vi "Test Get Named Ranges.vi"(11 "Test Case In":refnum<class "Test Open Xml.lvclass">) -> (0 "error out":errorcluster, 3 "Test Case Out":refnum<class "Test Open Xml.lvclass">)   [LabVIEW 2020, in "Test Open Xml.lvclass"]
uses:
  Test Open Xml.lvclass
  C:/Program Files/National Instruments/LabVIEW 2025/vi.lib/Astemes/LUnit/Test Case.lvclass
  Source/Cell DataType.ctl
  <vilib>/Astemes/LUnit/Test Case.lvclass/Test Case.ctl
  75fec585-59d7-4050-a2b8-3c2cca1562a1.vi
  c842f118-240e-4daf-a2da-7e37ae4209a2.vi
  f6172169-f5fa-494e-af90-d316b3356897.vi
  a79cc3df-4eee-4479-a611-92cfecdf73e7.vi
  c842f118-240e-4daf-a2da-7e37ae4209a2.vi/492de82e-1417-411c-9e2f-039d34dd0f56.vi
  Source/Excel Cell Address to Numeric Indices.vi
  Source/Numeric Indices to Excel Cell Address.vi
  c842f118-240e-4daf-a2da-7e37ae4209a2.vi/b0ca85c4-5697-48fb-9b3b-38ca6a246b1e.vi
  <vilib>/Astemes/LUnit/Append Fail Result.vi
  <vilib>/Astemes/LUnit/Append Pass Result.vi
  <vilib>/Astemes/LUnit/Run In UI.vi
  <vilib>/Utility/error.llb/Clear Errors.vi
  Source/Get WorksheetPart.vi
  Source/Get or Add Cell.vi
  Source/Create CellValue.vi
  Source/Set CellValue.vi
  Source/Set Cell DataType.vi
  Source/Open Xml.lvlib
  <vilib>/Astemes/LUnit/Test Case.lvclass
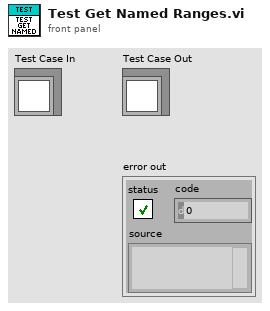
[diagram p1: front panel]
types:
  T1 = enum16{"Boolean", "Numeric", "String", "String2", "Array"}
  T2 = enum16{"Boolean", "Numeric", "String", "String2", "Array"}[]
  T3 = typedef "Open Xml.lvlib/Cell DataType.ctl" = enum16{"Void", "Boolean", "Number", "Error", "SharedString", "String", "InlineString", "Date"}
  T4 = cluster{"Number":dbl, "String":string, "Boolean":bool, "Timestamp":timestamp, "Error":errorcluster}
  T5 = cluster{"Number":dbl, "String":string, "Boolean":bool, "Time Stamp":timestamp, "Error":errorcluster}[][]
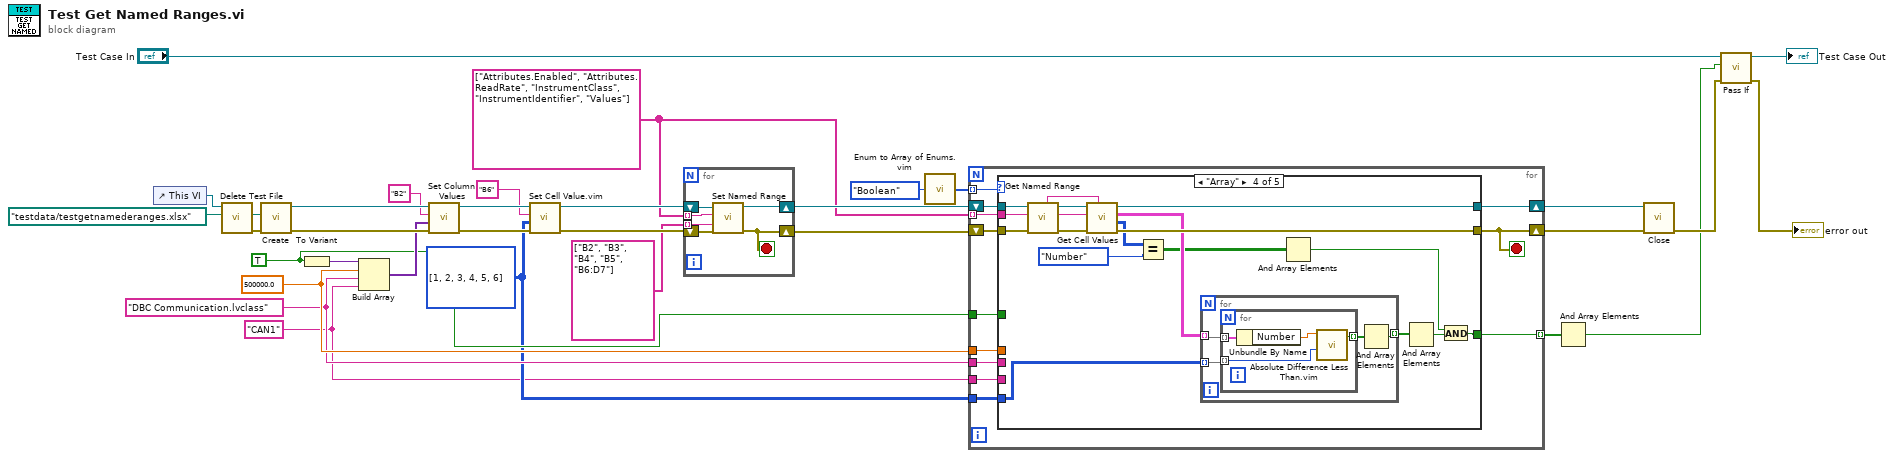
[diagram p0: block diagram]
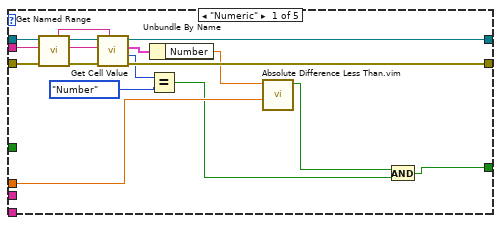
[diagram p2: hidden frame]
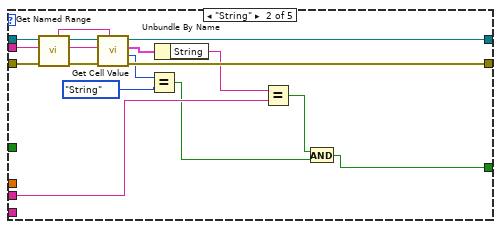
[diagram p3: hidden frame]
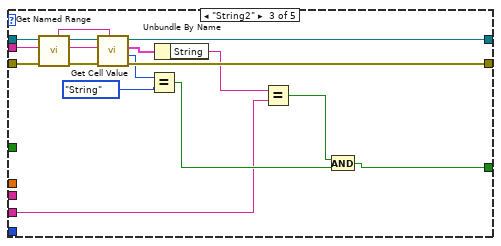
[diagram p4: hidden frame]
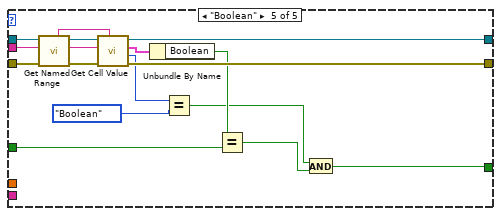
[diagram p5: hidden frame]
diagram:
  w4 = i32[][] [[1, 2, 3], [4, 5, 6]]
  w1 = "CAN1" ("element")
  w5 = "DBC Communication.lvclass"
  w7 = 500000.0
  w6 = TRUE
  w11 = string[] ["Attributes.Enabled", "Attributes.ReadRate", "InstrumentClass", "InstrumentIdentifier", "Values"] ("Range Names")
  n1 = control-ref of="This VI"() -> (w28:refnum<vi>)
  n2 = call "Delete Test File.vi"("name or relative path"=path "testdata/testgetnamederanges.xlsx", "VI in"=w28) -> ("error out"=w25:errorcluster, "deleted path"=w26:path)  [unwired: 8 in]
  n3 = call "Create.vi"("error in"=w25, "Path"=w26) -> ("error out"=w24:errorcluster, "SpreadsheetDoc"=w22:refnum<k24>)  [unwired: 8 in]
  n4 = To Variant(anything=w6) -> (Variant=w19:variant)
  n5 = Build Array(w19, w7, w5, w1) -> (w20:variant[])
  n6 = call "Set Column Values.vi"("error in"=w24, "Values"=w20, "Cell Address"="B2", "SpreadsheetDoc"=w22) -> ("error out"=w23:errorcluster, "SpreadsheetDoc out"=w16:refnum<k24>)  [unwired: 6 in]
  n7 = call "Set Cell Value.vim"("error in"=w23, "Value"=w4, "Cell Address"="B6", "SpreadsheetDoc in"=w16) -> ("error out"=w17:errorcluster, "SpreadsheetDoc out"=w15:refnum<k24>)  [unwired: 6 in]
  n8 = for {
    tunnel: w11 -> [w37] mode=indexing
    tunnel: string[] ["B2", "B3", "B4", "B5", "B6:D7"] ("Range Names") -> [w36] mode=indexing
    shift-right: [w35] -> w18
    shift-left: w17 -> [w39]
    shift-right: [w34] -> w12
    shift-left: w15 -> [w38]
    stop <- w35 stop-if-true
    n9 = call "Set Named Range.vi"("error in"=w39, "Cell Range"=w36, "Named Range Identifier"=w37, "SpreadsheetDoc in"=w38) -> ("error out"=w35:errorcluster, "SpreadsheetDoc out"=w34:refnum<k24>)  [unwired: 6 in]
  }
  n10 = call "Enum to Array of Enums.vim"("enum"=T1."Boolean") -> ("array of enums"=w8:T2)
  n11 = for {
    shift-right: [w47] -> w30
    shift-left: w18 -> [w51]
    tunnel: w11 -> [w50] mode=indexing
    shift-right: [w48] -> w10
    shift-left: w12 -> [w49]
    tunnel: w8 -> [w46] mode=indexing
    tunnel: w7 -> [w45]
    tunnel: w6 -> [w44]
    tunnel: w5 -> [w43]
    tunnel: w4 -> [w42]
    tunnel: [w41] -> w3 mode=indexing
    tunnel: w1 -> [w40]
    stop <- w47 stop-if-true
    n12 = case shown="\"Array\"" w46 {
      tunnel: w51 -> [w67 w84 w101 w119 w144]
      tunnel: w50 -> [w66 w83 w100 w118 w143]
      tunnel: w49 -> [w65 w82 w99 w117 w142]
      tunnel: [w64 w81 w98 w116 w141] -> w48
      tunnel: [w60 w77 w94 w112 w137] -> w47
      tunnel: w45 -> [w55 _ _ _ _]
      tunnel: w44 -> [_ _ _ _ w132]
      tunnel: w43 -> [_ w72 _ _ _]
      tunnel: w42 -> [_ _ _ w109 _]
      tunnel: [w52 w69 w87 w105 w129] -> w41
      tunnel: w40 -> [_ _ w86 _ _]
      frame "Numeric" {
        n13 = call "Get Named Range.vi"("error in"=w67, "Range Identifier"=w66, "SpreadsheetDoc in"=w65) -> ("error out"=w68:errorcluster, "Range"=w63:string, "SpreadsheetDoc out"=w62:refnum<k24>, "Sheet Name"=w61:string)  [unwired: 5 in]
        n14 = call "Get Cell Value.vi"("Sheet Name"=w61, "error in"=w68, "Cell Address"=w63, "SpreadsheetDoc in"=w62) -> ("error out"=w60:errorcluster, "Type"=w58:T3, "Cell Value"=w59:T4, "SpreadsheetDoc out"=w64:refnum<k24>)  [unwired: 4 in]
        n15 = Equal?(x=w58, y=Cell_DataType."Number") -> (x = y?=w54:bool)
        n16 = Unbundle By Name(w59) -> ("Number"=w56:dbl)
        n17 = call "Absolute Difference Less Than.vim"("Number 2"=w55, "Number 1"=w56) -> ("In Limit"=w53:bool)  [unwired: 9 in]
        n18 = And(x=w53, y=w54) -> (x .and. y?=w52:bool)
      }
      frame "String" {
        n19 = call "Get Named Range.vi"("error in"=w84, "Range Identifier"=w83, "SpreadsheetDoc in"=w82) -> ("error out"=w85:errorcluster, "Range"=w80:string, "SpreadsheetDoc out"=w79:refnum<k24>, "Sheet Name"=w78:string)  [unwired: 5 in]
        n20 = call "Get Cell Value.vi"("Sheet Name"=w78, "error in"=w85, "Cell Address"=w80, "SpreadsheetDoc in"=w79) -> ("error out"=w77:errorcluster, "Type"=w75:T3, "Cell Value"=w76:T4, "SpreadsheetDoc out"=w81:refnum<k24>)  [unwired: 4 in]
        n21 = Equal?(x=w75, y=Cell_DataType."String") -> (x = y?=w70:bool)
        n22 = Unbundle By Name(w76) -> ("String"=w73:string)
        n23 = Equal?(x=w73, y=w72) -> (x = y?=w71:bool)
        n24 = And(x=w71, y=w70) -> (x .and. y?=w69:bool)
      }
      frame "String2" {
        n25 = call "Get Named Range.vi"("error in"=w101, "Range Identifier"=w100, "SpreadsheetDoc in"=w99) -> ("error out"=w102:errorcluster, "Range"=w97:string, "SpreadsheetDoc out"=w96:refnum<k24>, "Sheet Name"=w95:string)  [unwired: 5 in]
        n26 = call "Get Cell Value.vi"("Sheet Name"=w95, "error in"=w102, "Cell Address"=w97, "SpreadsheetDoc in"=w96) -> ("error out"=w94:errorcluster, "Type"=w92:T3, "Cell Value"=w93:T4, "SpreadsheetDoc out"=w98:refnum<k24>)  [unwired: 4 in]
        n27 = Equal?(x=w92, y=Cell_DataType."String") -> (x = y?=w88:bool)
        n28 = Unbundle By Name(w93) -> ("String"=w90:string)
        n29 = Equal?(x=w90, y=w86) -> (x = y?=w89:bool)
        n30 = And(x=w89, y=w88) -> (x .and. y?=w87:bool)
      }
      frame "Array" {
        n31 = call "Get Named Range.vi"("error in"=w119, "Range Identifier"=w118, "SpreadsheetDoc in"=w117) -> ("error out"=w120:errorcluster, "Range"=w115:string, "SpreadsheetDoc out"=w114:refnum<k24>, "Sheet Name"=w113:string)  [unwired: 5 in]
        n32 = call "Get Cell Values.vi"("Sheet Name"=w113, "error in"=w120, "Cell Addresses"=w115, "SpreadsheetDoc in"=w114) -> ("error out"=w112:errorcluster, "Types"=w111:T3[][], "Cell Values"=w108:T5, "SpreadsheetDoc out"=w116:refnum<k24>)  [unwired: 4 in]
        n33 = Equal?(x=w111, y=Cell_DataType."Number") -> (x = y?=w104:bool[][])
        n34 = for {
          tunnel: w109 -> [w124] mode=indexing
          tunnel: w108 -> [w123] mode=indexing
          tunnel: [w121] -> w107 mode=indexing
          n35 = for {
            tunnel: w124 -> [w126] mode=indexing
            tunnel: w123 -> [w128] mode=indexing
            tunnel: [w125] -> w122 mode=indexing
            n36 = Unbundle By Name(w128) -> ("Number"=w127:dbl)
            n37 = call "Absolute Difference Less Than.vim"("Number 2"=w126, "Number 1"=w127) -> ("In Limit"=w125:bool)  [unwired: 9 in]
          }
          n38 = And Array Elements(Boolean array=w122) -> (logical AND=w121:bool)
        }
        n39 = And Array Elements(Boolean array=w104) -> (logical AND=w103:bool)
        n40 = And Array Elements(Boolean array=w107) -> (logical AND=w106:bool)
        n41 = And(x=w103, y=w106) -> (x .and. y?=w105:bool)
      }
      frame "Boolean" {
        n42 = call "Get Named Range.vi"("error in"=w144, "Range Identifier"=w143, "SpreadsheetDoc in"=w142) -> ("error out"=w145:errorcluster, "Range"=w140:string, "SpreadsheetDoc out"=w139:refnum<k24>, "Sheet Name"=w138:string)  [unwired: 5 in]
        n43 = call "Get Cell Value.vi"("Sheet Name"=w138, "error in"=w145, "Cell Address"=w140, "SpreadsheetDoc in"=w139) -> ("error out"=w137:errorcluster, "Type"=w135:T3, "Cell Value"=w136:T4, "SpreadsheetDoc out"=w141:refnum<k24>)  [unwired: 4 in]
        n44 = Unbundle By Name(w136) -> ("Boolean"=w133:bool)
        n45 = Equal?(x=w135, y=Cell_DataType."Boolean") -> (x = y?=w130:bool)
        n46 = Equal?(x=w133, y=w132) -> (x = y?=w131:bool)
        n47 = And(x=w130, y=w131) -> (x .and. y?=w129:bool)
      }
    }
  }
  n48 = And Array Elements(Boolean array=w3) -> (logical AND=w2:bool)
  n49 = call "Close.vi"("error in"=w30, "SpreadsheetDoc"=w10) -> ("error out"=w29:errorcluster)  [unwired: 9 in]
  n50 = call <vilib>:"Pass If.vi"("error in (no error)"=w29, "Pass?"=w2, "LUnit Test Case In"="Test Case In") -> ("error out"=→"error out":errorcluster, "LUnit Test Case Out"=→"Test Case Out":refnum<class "Test Open Xml.lvclass">)  [unwired: 7 in]
